vi "Logic_Export_Raw_Mixed_Signal_to_CSV.vi"(4 "Analog Downsample Ratio":i32=1, 6 "Enabled Analog Channels":i32[](array[numeric]), 8 "error in (no error)":errorcluster, 9 "Enabled Digital Channels":i32[](array[numeric]), 10 "Filepath Input":string, 11 "Session Ref In":T1) -> (0 "error out":errorcluster, 3 "Session Ref Out":T1)   [LabVIEW 2023]
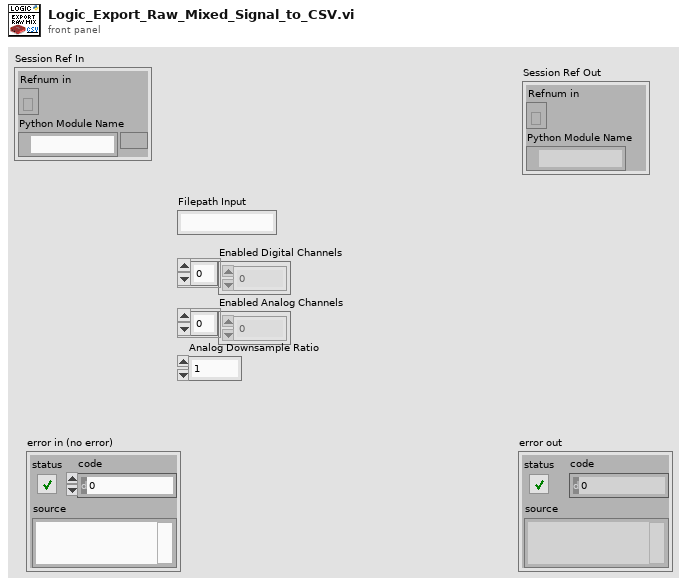
[diagram p1: front panel]
types:
  T1 = cluster{"Refnum in":refnum<k35>, "Python Module Name":path}
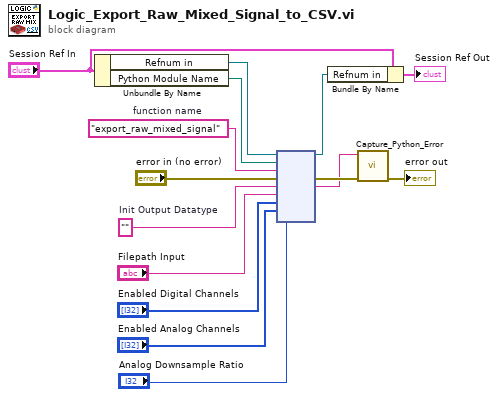
[diagram p0: block diagram]
diagram:
  w14 = "export_raw_mixed_signal"  # function name
  w13 = ""  # Init Output Datatype
  n1 = Unbundle By Name("Session Ref In") -> ("Refnum in"=w12:refnum<k35>, "Python Module Name"=w11:path)
  n2 = node(w12, w11, w14, "error in (no error)", w13, "Filepath Input", "Enabled Digital Channels", "Enabled Analog Channels", "Analog Downsample Ratio") -> (w9:refnum<k35>, w3:errorcluster, w1:string)  [unwired: 4 in, 2 out]
  n3 = Bundle By Name(cluster="Session Ref In", "Refnum in"=w9) -> (→"Session Ref Out":T1)
  n4 = call "Capture_Python_Error.vi"("error in (no error)"=w3, "Error Message (start with ERROR)"=w1) -> ("error out"=→"error out":errorcluster)  [unwired: 9 in]
